vi "GUI_laptop v11g2.vi"() -> ()   [LabVIEW 2019]
uses:
  <vilib>/Math Plots/3D Math Plots/3D Scatter/3D Scatter XCtrl/3D Scatter.xctl
  <vilib>/Platform/TimedLoop/XDataNode/timing_clust.ctl
  <vilib>/Platform/TimedLoop/XDataNode/nitl_modes.ctl
  <vilib>/Platform/TimedLoop/XDataNode/wakeup.ctl
  <vilib>/Analysis/_algsub.llb/Real Vector Norm.vi
  <vilib>/Instr/_visa.llb/VISA Configure Serial Port (Instr).vi
  <vilib>/Utility/file.llb/Write Delimited Spreadsheet (DBL).vi
  <vilib>/addons/System Identification/Data Preprocess.llb/SI Lowpass Filter (MISO Array).vi
  <vilib>/Math Plots/3D Math Plots/3D Scatter/3D Scatter Datatype/Public/Plot Helper (Vector).vi
  <vilib>/platform/TimedLoop/XDataNode/XDataNode.xnode
  <vilib>/Platform/TimedLoop/XDataNode/XDNodeRunTimeDep.lvlib
  <vilib>/Analysis/NI_AALPro.lvlib
  <vilib>/Math Plots/3D Math Plots/3D Scatter/3D Scatter Datatype/3D Scatter Datatype.lvclass
  <vilib>/addons/System Identification/NI_SysID.lvlib
panel:
  in  "l3_init":dbl=2.0
  in  "Motion scale L3 outside rcm":dbl=2.0
  in  "L5 Deadzone":dbl
  in  "Sample rate":u32=500
  in  "Cutoff Frequency":dbl=10.0
  in  "Motion scale L1 L2":dbl=10.0
  in  "Motion scale L3":dbl=2.0
  in  "Save Path 4":path=path "C:/Users/jimmy/Documents/GitHub/Arduino-LabVIEW/zhantao/read_data_abs_filtered.csv"
  in  "Save Path 3":path=path "C:/Users/jimmy/Documents/GitHub/Arduino-LabVIEW/zhantao/read_data_abs_sending.csv"
  out "stimulus signals out":dbl[][](array[numeric]) format="%.2f"
  in  "L5 Offset":dbl
  in  "L5 Scale":dbl=1.0
  in  "Motion Scale L4":dbl=30.0
  out "spreadsheet string":string
  in  "Save Path 2":path=path "C:/Users/jimmy/Documents/GitHub/Arduino-LabVIEW/zhantao/read_data_delt.csv"
  out "send values":dbl[](array[numeric])
  out "Robot Feedback (l1 l2 l3 l4)":dbl[](array[numeric])
  in  "UDP Send":bool
  in  "UDP Recv":bool
  in  "L5 bound":dbl=1000.0
  in  "L4 bound (deg)":dbl=1000.0
  in  "L3 bound (mm)":dbl=1000.0
  in  "L2 bound (deg)":dbl=1000.0
  in  "L1 bound (deg)":dbl=1000.0
  in  "Joystick Type":dbl(ring)=1.0 items=["Rigid Joystick", "Free Joystick"]
  out "Finished Late? [i-1]":bool
  in  "Epsilon":dbl=0.2
  out "3D Scatter":refnum<class "3D Plot Datatype.lvclass">[](xcontrol)
  out "Random Point":dbl[](array[numeric])
  out "Virtual Cursor":dbl[](array[numeric])
  out "Iteration Duration":i64
  in  "Num of Points":i32=10
  in  "z bound":dbl=2.0
  in  "y bound":dbl=5.0
  in  "x bound":dbl=5.0
  in  "Stop":bool
  in  "Round Decimals":dbl=2.0 format="%#_15g"
  in  "Save Data":bool
  in  "Save Path":path=path "C:/Users/jimmy/Documents/GitHub/Arduino-LabVIEW/zhantao/read_data_abs.csv"
  in  "x speed":dbl=0.5
  in  "z speed":dbl=0.5
  in  "y speed":dbl=0.5
  out "error out":errorcluster
  in  "baud rate":u32=250000
  in  "VISA resource name":refnum<visa-resource-name>
  # "Joystick Selection"
  # "Plotting"
  # "Data Saving"
  # "Arduino Communication"
  # "Master Slave Communication"
  # "Parameters"
  # "TODO: add a lowpass filter for l5"
  # "TODO: fix the bounds; currently bounds are arbitrary"
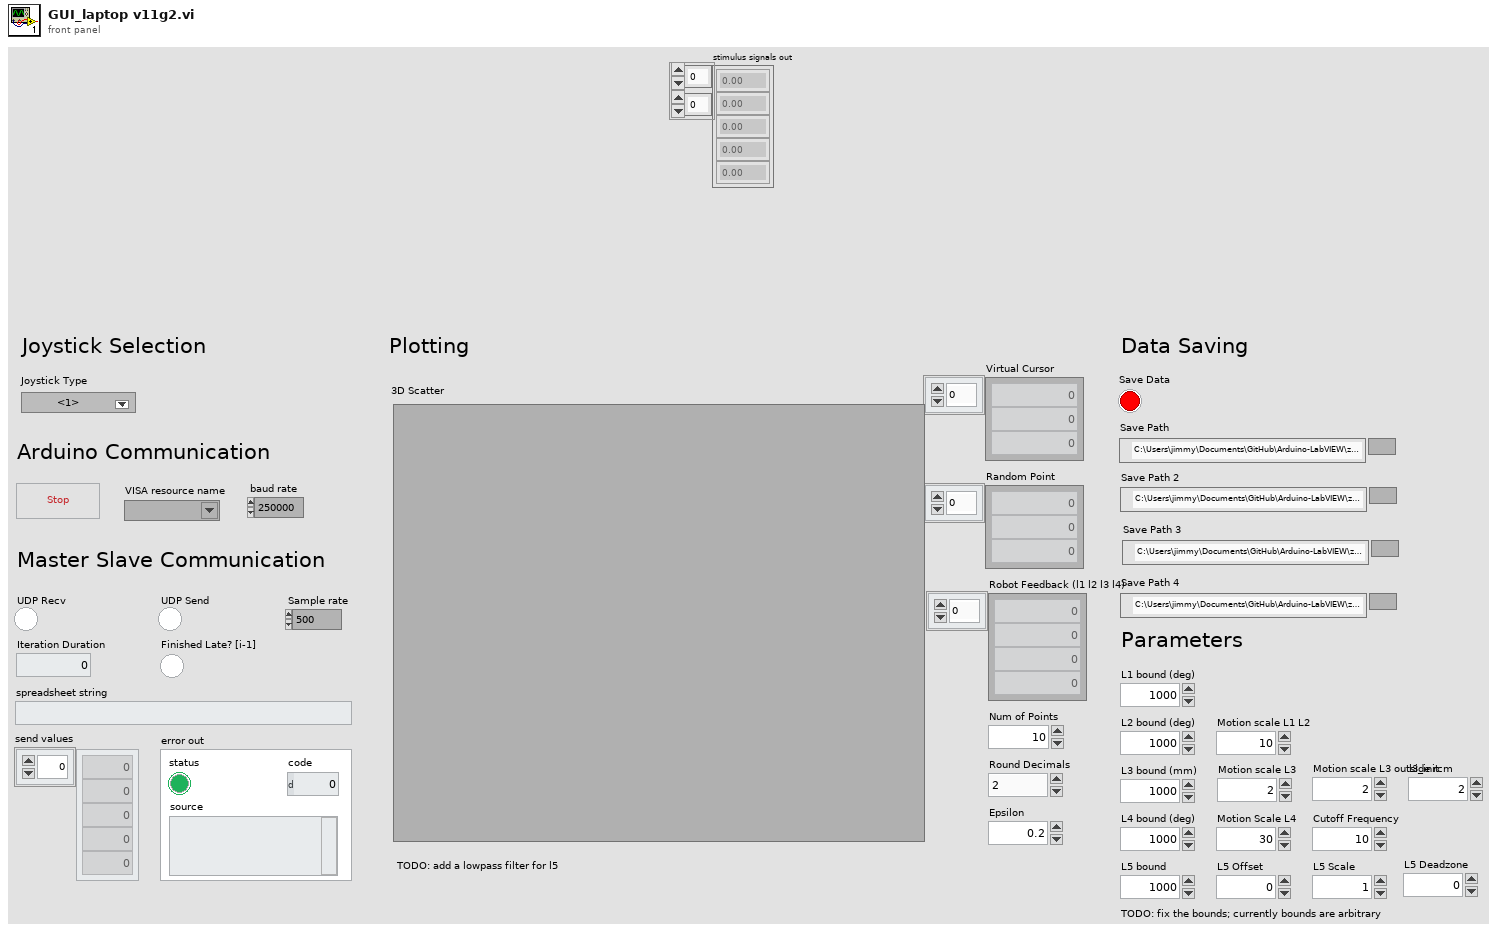
[diagram p1: front panel]
types:
  T1 = typedef "XDNodeRunTimeDep.lvlib/timing_clust.ctl" = cluster{"Expected End [f-1]":u64, "Actual End [f-1]":u64, "Finished Late? [f-1]":bool, "Expected End [i-1]":u64, "Actual End [i-1]":u64, "Finished Late? [i-1]":bool, "Expected Start [i]":u64, "Actual Start [i]":u64, "Expected Start [f]":u64, "Actual Start [f]":u64, "Source Name":string, "Structure Name":string, "Period":i64, "Deadline":i64, "Offset":i64, "Start":i64, "Priority":i32, "Timeout":i32, "Mode":T2, "Wakeup Reason":T3, "Error":errorcluster, "Source Type":string, "Secondary Source Type":string, "Global End Time":u64, "Global Start Time":u64, "Frame Duration":u64, "Iteration Duration":u64, "Assigned CPU":i32, "I/O Scan Engine Mode":u32}
  T2 = typedef "XDNodeRunTimeDep.lvlib/nitl_modes.ctl" = enum32{"No Change", "Process missed periods, maintain original phase", "Discard missed periods, maintain original phase", "Process missed periods, ignore original phase", "Discard missed periods, ignore original phase"}
  T3 = typedef "XDNodeRunTimeDep.lvlib/wakeup.ctl" = enum32{"Normal", "Aborted", "Asynchronous wakeup", "Timing source error", "Timed loop error", "Timeout"}
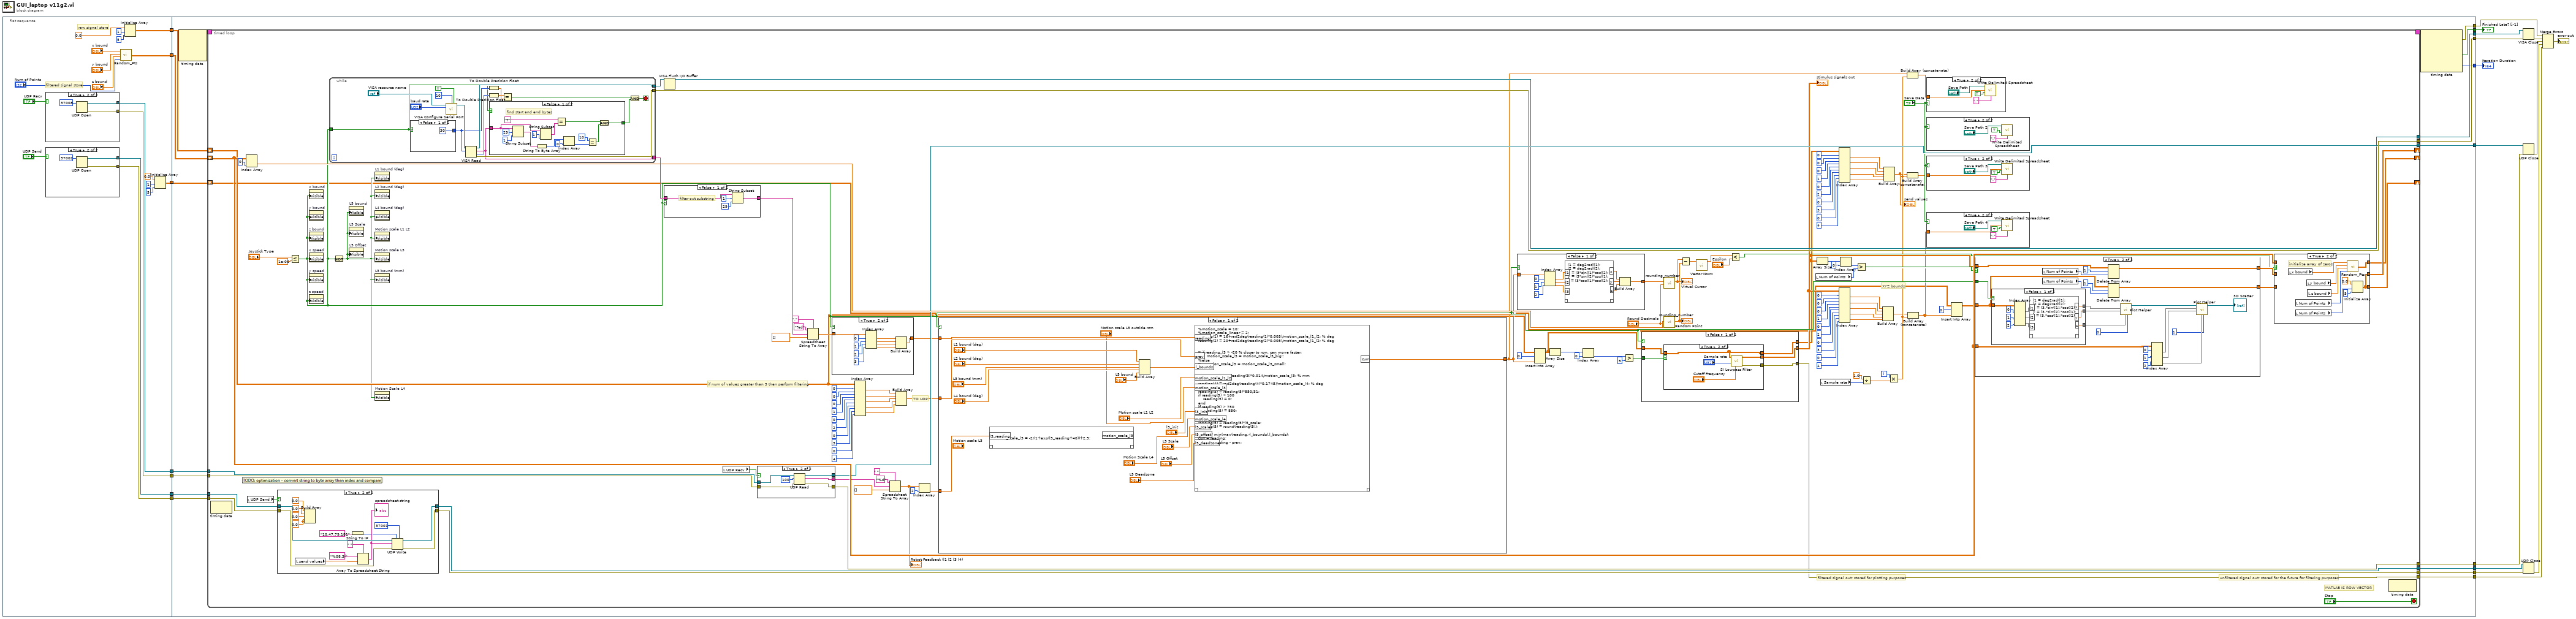
[diagram p0: block diagram]
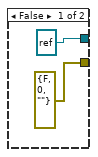
[diagram p2: hidden frame]
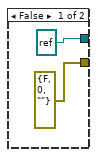
[diagram p3: hidden frame]
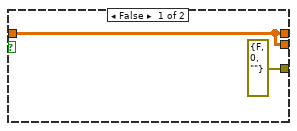
[diagram p6: hidden frame]
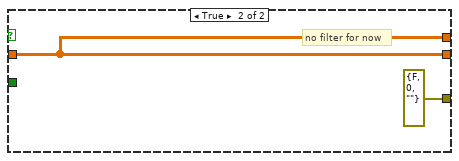
[diagram p7: hidden frame]
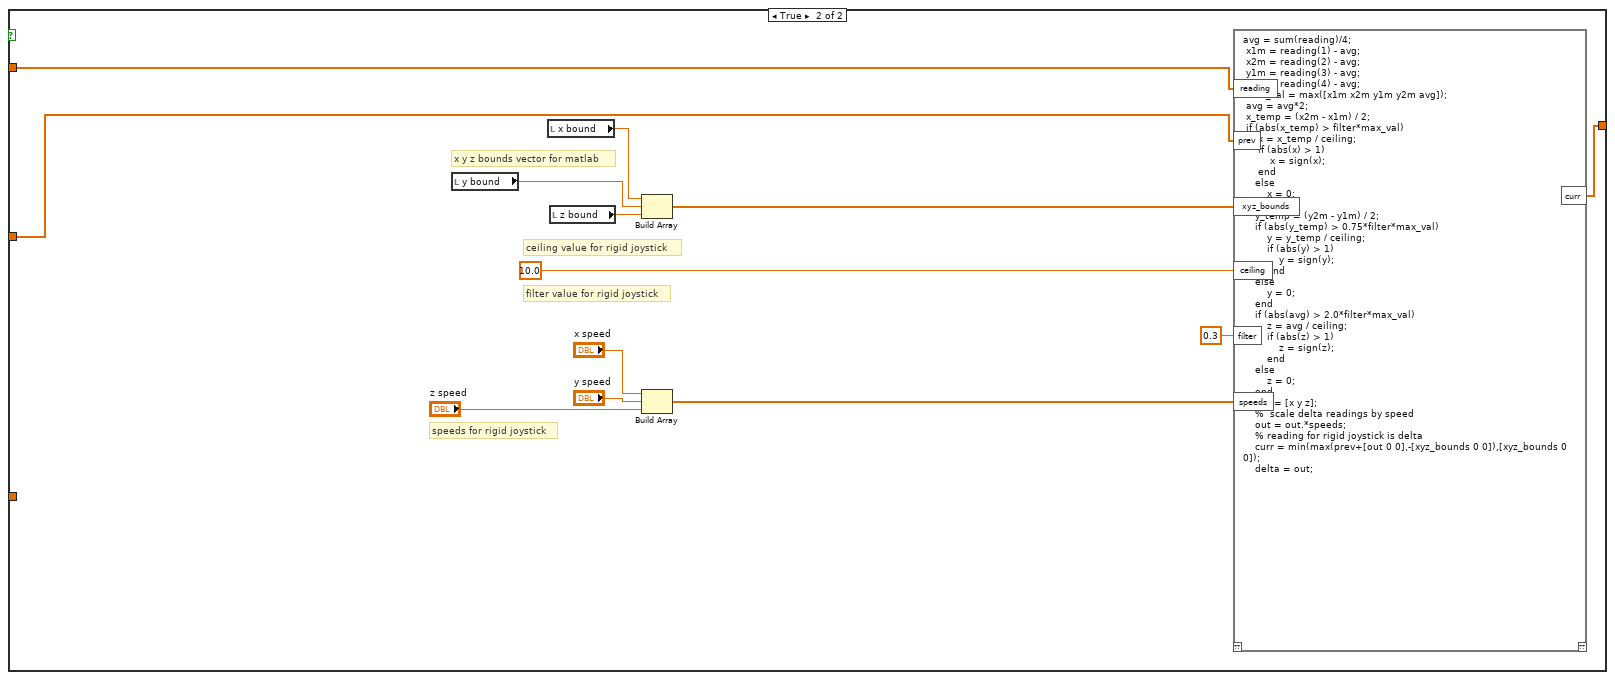
[diagram p8: hidden frame]
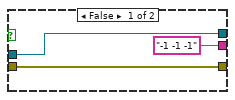
[diagram p11: hidden frame]
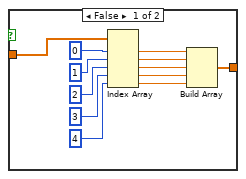
[diagram p15: hidden frame]
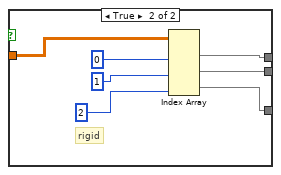
[diagram p18: hidden frame]
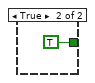
[diagram p19: hidden frame]
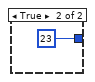
[diagram p20: hidden frame]
diagram:
  n1 = flat-sequence {
    tunnel: [w32] -> w17
    tunnel: [w36] -> w16
    tunnel: [w31] -> w15
    tunnel: [w30] -> w14
    tunnel: [w27] -> w13
    tunnel: [w26] -> w12
    tunnel: [w22] -> w1
    tunnel: [w67] -> w21
    tunnel: [w66] -> w20
    tunnel: [w64] -> w11
    tunnel: [w62] -> w19
    tunnel: [w61] -> w18
    tunnel: w17 -> [w65]
    tunnel: w16 -> [w63]
    tunnel: w15 -> [w60]
    tunnel: w14 -> [w59]
    tunnel: w13 -> [w58]
    tunnel: w12 -> [w57]
    tunnel: [w56] -> w5
    tunnel: [w55] -> w10
    tunnel: [w54] -> w4
    tunnel: [w53] -> w3
    tunnel: [w52] -> w2
    tunnel: w1 -> [w51]
    frame #0 {
      # "filtered signal store"
      # "raw signal store"
      n2 = case shown="True" "UDP Recv" {
        tunnel: [refnum<k16> refnum ("port") w49] -> w30
        tunnel: [errorcluster {"status"=FALSE, "code"=0, "source"=""} ("error out") w48] -> w27
        frame False {
        }
        frame True {
          n3 = UDP Open(11:u16 37008 ("port")) -> (port=w49:refnum<k16>, 0:w48:errorcluster)  [unwired: 4 in, 1 out]
        }
      }
      n4 = case shown="True" "UDP Send" {
        tunnel: [refnum<k16> refnum ("port") w44] -> w31
        tunnel: [errorcluster {"status"=FALSE, "code"=0, "source"=""} ("error out") w43] -> w26
        frame False {
        }
        frame True {
          n5 = UDP Open(11:u16 37002 ("port")) -> (port=w44:refnum<k16>, 0:w43:errorcluster)  [unwired: 4 in, 1 out]
        }
      }
      n6 = call "Random_Pts.vi"("Num of Points"="Num of Points", "z bound"="z bound", "y bound"="y bound", "x bound"="x bound") -> ("appended array"=w36:dbl[][])
      n7 = Initialize Array(0.0 ("element"), 1 ("dimension size"), 5 ("dimension size")) -> (w32:dbl[][])
      n8 = Initialize Array(0.0 ("element"), 1 ("dimension size"), 5 ("dimension size")) -> (w22:dbl[][])
    }
    frame #1 {
      n9 = node-c288() -> (w69:T1)  [unwired: 4 in]
      n10 = timed-loop {
        tunnel: [w137] -> w67
        tunnel: [w193] -> w66
        shift-right: [w192] -> _
        shift-left: w65 -> [w91]
        timing: w69 -> [_]
        timing-out: [_] -> w68
        shift-right: [w188] -> _
        shift-left: w63 -> [w189]
        tunnel: w60 -> [w151]
        tunnel: w59 -> [w150]
        tunnel: w58 -> [w148]
        tunnel: w57 -> [w147]
        tunnel: [w146] -> w56
        tunnel: [w145] -> w55
        tunnel: [w144] -> w54
        tunnel: [w143] -> w53
        tunnel: [w126] -> w52
        shift-right: [w82] -> _
        shift-left: w51 -> [w85]
        i -> [w80]
        stop <- "Stop" stop-if-true
        # "unfiltered signal out; stored for the future for filtering purposes"
        # "filtered signal out; stored for plotting purposes"
        # "XYZ bounds"
        # "if num of values greater than 5 then perform filtering"
        # "TO UDP"
        # "MATLAB IS ROW VECTOR"
        n11 = node-c288() -> ()  [unwired: 1 in, 1 out]
        n12 = Index Array(array=w189, index (col)=0 ("index (row)")) -> (element=w160:dbl[])  [unwired: 1 in]
        n13 = local read "UDP Send"() -> (w75:bool)
        n14 = case shown="True" w75 {
          tunnel: w151 -> [w250 w266]
          tunnel: w147 -> [w251 w262]
          tunnel: [w251 w258] -> w145
          tunnel: [w250 w257] -> w143
          frame False {
          }
          frame True {
            w256 = 0.0 ("element")
            n15 = local read "send values"() -> (w252:dbl[])
            n16 = Build Array(0.0 ("element"), 0.0 ("element"), 0.0 ("element"), w256, w256) -> ()  [unwired: 1 out]
            n17 = String To IP(1:"10.47.79.181" ("name")) -> (0:w260:u32)
            n18 = Array To Spreadsheet String(delimiter (Tab)=" ", array=w252, 3:"%08.3f" ("format string")) -> (spreadsheet string=w263:string)
            "spreadsheet string" <- w263
            n19 = UDP Write(address=w260, port or service name=u16 37001, connection ID=w266, data in=w263, 8:w262) -> (error out=w258:errorcluster, 3:w257:refnum<k16>)  [unwired: 1 in]
          }
        }
        n20 = Less Or Equal?(x="Joystick Type", y=1e-06) -> (x <= y?=w127:bool)
        n21 = property on="x bound" class="DigNum (strict)"("Visible"=w127) -> ()  [unwired: 2 in, 2 out]
        n22 = property on="y bound" class="DigNum (strict)"("Visible"=w127) -> ()  [unwired: 2 in, 2 out]
        n23 = property on="z bound" class="DigNum (strict)"("Visible"=w127) -> ()  [unwired: 2 in, 2 out]
        n24 = property on="x speed" class="DigNum (strict)"("Visible"=w127) -> ()  [unwired: 2 in, 2 out]
        n25 = property on="y speed" class="DigNum (strict)"("Visible"=w127) -> ()  [unwired: 2 in, 2 out]
        n26 = property on="z speed" class="DigNum (strict)"("Visible"=w127) -> ()  [unwired: 2 in, 2 out]
        n27 = while {
          tunnel: [w373] -> w162
          tunnel: [w386] -> w193
          tunnel: [w380] -> w138
          tunnel: w127 -> [w374]
          stop <- w376 stop-if-true
          n28 = case shown="False" w374 {
            tunnel: [30 u32 23 ("byte count")] -> w379
            frame False {
            }
            frame True {
            }
          }
          n29 = call-poly "VISA Configure Serial Port"("VISA resource name"="VISA resource name", "termination char\n(0xA = '\\n' = LF)"=u8 10 ("termination char\n(0xA = '\\n' = LF)"), "Enable Termination\nChar (T)"=TRUE ("Enable Termination\nChar (T)"), "baud rate (9600)"="baud rate") -> ("VISA resource name out"=w381:refnum<visa-resource-name>)  [unwired: 10 in, 1 out]
          n30 = VISA Read(VISA resource name=w381, byte count=w379) -> (VISA resource name out=w380:refnum<visa-resource-name>, read buffer=w373:string, return count=w388:u32, error out=w386:errorcluster)  [unwired: 1 in]
          n31 = To Double Precision Float(number=w379) -> (double precision float=w378:dbl)
          n32 = To Double Precision Float(number=w388) -> (double precision float=w387:dbl)
          n33 = case shown="False" w374 {
            tunnel: [w395 TRUE] -> w375
            tunnel: w373 -> [w398 _]
            frame False {
              # "find start and end bytes"
              n34 = String Subset(string=w398, offset (0)=29, length (rest)=1) -> (substring=w393:string)
              n35 = String To Byte Array(string=w393) -> (unsigned byte array=w392:u8[])
              n36 = String Subset(string=w398, length (rest)=1) -> (substring=w401:string)  [unwired: 1 in]
              n37 = Equal?(x="T", y=w401) -> (x = y?=w397:bool)
              n38 = Index Array(array=w392, index=0) -> (element=w390:u8)
              n39 = Equal?(x=10, y=w390) -> (x = y?=w396:bool)
              n40 = And(x=w397, y=w396) -> (x .and. y?=w395:bool)
            }
            frame True {
            }
          }
          n41 = Equal?(x=w387, y=w378) -> (x = y?=w377:bool)
          n42 = And(x=w377, y=w375) -> (x .and. y?=w376:bool)
        }
        n43 = Not(x=w127) -> (.not. x?=w89:bool)
        n44 = property on="L5 bound" class="DigNum (strict)"("Visible"=w89) -> ()  [unwired: 2 in, 2 out]
        n45 = property on="L5 Scale" class="DigNum (strict)"("Visible"=w89) -> ()  [unwired: 2 in, 2 out]
        n46 = property on="L5 Offset" class="DigNum (strict)"("Visible"=w89) -> ()  [unwired: 2 in, 2 out]
        n47 = property on="L1 bound (deg)" class="DigNum (strict)"("Visible"=w89) -> ()  [unwired: 2 in, 2 out]
        n48 = property on="L2 bound (deg)" class="DigNum (strict)"("Visible"=w89) -> ()  [unwired: 2 in, 2 out]
        n49 = property on="L4 bound (deg)" class="DigNum (strict)"("Visible"=w89) -> ()  [unwired: 2 in, 2 out]
        n50 = property on="Motion scale L1 L2" class="DigNum (strict)"("Visible"=w89) -> ()  [unwired: 2 in, 2 out]
        n51 = property on="Motion scale L3" class="DigNum (strict)"("Visible"=w89) -> ()  [unwired: 2 in, 2 out]
        n52 = property on="L3 bound (mm)" class="DigNum (strict)"("Visible"=w89) -> ()  [unwired: 2 in, 2 out]
        n53 = property on="Motion Scale L4" class="DigNum (strict)"("Visible"=w89) -> ()  [unwired: 2 in, 2 out]
        n54 = VISA Flush I/O Buffer(VISA resource name=w138) -> (VISA resource name out=w137:refnum<visa-resource-name>)  [unwired: 2 in, 1 out]
        n55 = case shown="False" w127 {
          tunnel: w162 -> [w295 w296]
          tunnel: [w292 w296] -> w161
          frame False {
            # "filter out substring"
            n56 = String Subset(string=w295, offset (0)=1, length (rest)=29) -> (substring=w292:string)
          }
          frame True {
          }
        }
        n57 = local read "UDP Recv"() -> (w149:bool)
        n58 = case shown="True" w149 {
          tunnel: w150 -> [w268 w275]
          tunnel: w148 -> [w269 w274]
          tunnel: [w269 w273] -> w146
          tunnel: [w268 w272] -> w144
          tunnel: ["-1 -1 -1" w270] -> w139
          frame False {
          }
          frame True {
            n59 = UDP Read(connection ID=w275, max size (548)=100, 8:w274) -> (data out=w270:string, error out=w273:errorcluster, 3:w272:refnum<k16>)  [unwired: 1 in, 2 out]
          }
        }
        n60 = Spreadsheet String To Array(delimiter (Tab)=",", format string="%d", spreadsheet string=w161, array type (2D Dbl)=dbl[] []) -> (array=w163:dbl[])
        n61 = case shown="True" w127 {
          tunnel: w163 -> [w297 w312]
          tunnel: [w302 w311] -> w135
          frame False {
            n62 = Index Array(array=w297, index #1=0 ("Plot ID"), index #2=1 ("Plot ID"), index #3=2 ("Plot ID"), index #4=3 ("Plot ID"), index #5=4 ("Plot ID")) -> (element #1=w305:dbl, element #2=w304:dbl, element #3=w303:dbl, element #4=w299:dbl, element #5=w298:dbl)
            n63 = Build Array(w305, w304, w303, w299, w298) -> (w302:dbl[])
          }
          frame True {
            n64 = Index Array(array=w312, index #1=0 ("Plot ID"), index #2=1 ("Plot ID"), index #3=2 ("Plot ID"), index #4=3 ("index")) -> (element #1=w315:dbl, element #2=w314:dbl, element #3=w313:dbl, element #4=w309:dbl)
            n65 = Build Array(w315, w314, w313, w309) -> (w311:dbl[])
          }
        }
        n66 = Index Array(array=w91, index (row) #1=0 ("disabled index (row)"), index (col) #1=0 ("disabled index (col)"), index (row) #2=0 ("disabled index (row)"), index (col) #2=1 ("disabled index (col)"), index (row) #3=0 ("disabled index (row)"), index (col) #3=2 ("disabled index (col)"), index (row) #4=0 ("disabled index (row)"), index (col) #4=3 ("disabled index (col)"), index (row) #5=0 ("disabled index (row)"), index (col) #5=4 ("disabled index (col)")) -> (element #1=w174:dbl, element #2=w173:dbl, element #3=w172:dbl, element #4=w165:dbl, element #5=w164:dbl)
        n67 = Spreadsheet String To Array(delimiter (Tab)=" ", format string="%d", spreadsheet string=w139, array type (2D Dbl)=dbl[] []) -> (array=w72:dbl[])
        "Robot Feedback (l1 l2 l3 l4)" <- w72
        n68 = Build Array(w174, w173, w172, w165, w164) -> (w136:dbl[])
        n69 = Index Array(array=w72, index=2) -> (element=w70:dbl)
        n70 = case shown="False" w127 {
          tunnel: w136 -> [w225 w236]
          tunnel: w135 -> [w226 w235]
          tunnel: [w224 w234] -> w110
          tunnel: w70 -> [w218 _]
          frame False {
            n71 = script code="motion_scale_l3 = -2/(1+exp(l3_reading+40))+2.5;"("l3_reading"=w218) -> ()  [unwired: 1 in, 2 out]
            n72 = Build Array("L1 bound (deg)", "L2 bound (deg)", "L3 bound (mm)", "L4 bound (deg)", "L5 bound") -> (w227:dbl[])
            n73 = script code="%motion_scale = 10;\n%motion_scale_linear = 2;\nreading(1) = 16+rad2deg(reading(1)*0.005)/motion_scale_l1_l2; % deg\nreading(2) = 20+rad2deg(reading(2)*0.005)/motion_scale_l1_l2; % deg\n\n\n%if reading_l3 > -20 % closer to rcm, can move faster;\n%    motion_scale_l3 = motion_scale_l3_big;;\n%else\n%   motion_scale_l3 = motion_scale_l3_small;\n%end\n\nreading(3) = -40-reading(3)*0.014/motion_scale_l3; % mm\n\nreading(4) = rad2deg(reading(4)*0.1745)/motion_scale_l4; % deg\n\nreading(5) = reading(5)*850/31;\nif reading(5) < 100\n    reading(5) = 0;\nend\nif reading(5) > 750\n    reading(5) = 850;\nend\n\nreading(5) = reading(5)*l5_scale;\nreading(5) = round(reading(5));\n\n%curr = min(max(reading,-l_bounds),l_bounds);\ncurr = reading;\ndelta = reading - prev;"("l_bounds"=w227, "motion_scale_l4"="Motion Scale L4", "reading"=w226, "prev"=w225, "l5_scale"="L5 Scale", "l5_offset"="L5 Offset", "motion_scale_l3"="Motion scale L3 outside rcm", "motion_scale_l1_l2"="Motion scale L1 L2", "l5_deadzone"="L5 Deadzone", "l3_init"="l3_init") -> ("curr"=w224:dbl[])  [unwired: 1 in, 1 out]
          }
          frame True {
            # "ceiling value for rigid joystick"
            # "filter value for rigid joystick"
            # "speeds for rigid joystick"
            # "x y z bounds vector for matlab"
            n74 = local read "y bound"() -> (w245:dbl)
            n75 = local read "x bound"() -> (w244:dbl)
            n76 = local read "z bound"() -> (w246:dbl)
            n77 = Build Array(w244, w245, w246) -> (w237:dbl[])
            n78 = Build Array("x speed", "y speed", "z speed") -> (w240:dbl[])
            n79 = script code="avg = sum(reading)/4;\n x1m = reading(1) - avg;\n x2m = reading(2) - avg;\n y1m = reading(3) - avg;\n y2m = reading(4) - avg;\n max_val = max([x1m x2m y1m y2m avg]);\n avg = avg*2;\n x_temp = (x2m - x1m) / 2;\n if (abs(x_temp) > filter*max_val)\n     x = x_temp / ceiling;\n     if (abs(x) > 1)\n         x = sign(x);\n     end\n    else\n        x = 0;\n    end\n    y_temp = (y2m - y1m) / 2;\n    if (abs(y_temp) > 0.75*filter*max_val)\n        y = y_temp / ceiling;\n        if (abs(y) > 1)\n            y = sign(y);\n        end\n    else\n        y = 0;\n    end\n    if (abs(avg) > 2.0*filter*max_val)\n        z = avg / ceiling;\n        if (abs(z) > 1)\n            z = sign(z);\n        end\n    else\n        z = 0;\n    end\n    out = [x y z];\n    %  scale delta readings by speed\n    out = out.*speeds;\n    % reading for rigid joystick is delta\n    curr = min(max(prev+[out 0 0],-[xyz_bounds 0 0]),[xyz_bounds 0 0]);\n    delta = out;"("xyz_bounds"=w237, "ceiling"=10.0 ("Real"), "filter"=0.3 ("Real"), "speeds"=w240, "reading"=w235, "prev"=w236) -> ("curr"=w234:dbl[])  [unwired: 1 in, 1 out]
          }
        }
        n80 = case shown="False" w127 {
          tunnel: [w323 w330] -> w190
          tunnel: w110 -> [w322 w330]
          frame False {
            n81 = Index Array(array=w322, index #1=0 ("Plot ID"), index #2=1 ("Plot ID"), index #3=2 ("Plot ID")) -> (element #1=w321:dbl, element #2=w320:dbl, element #3=w319:dbl)
            n82 = script code="l1 = deg2rad(l1);\nl2 = deg2rad(l2);\nx = l3*sin(l1)*cos(l2);\ny = l3*sin(l2)*cos(l1);\nz = l3*cos(l1)*cos(l2);"("l1"=w321, "l2"=w320, "l3"=w319) -> ("x"=w326:dbl, "y"=w325:dbl, "z"=w324:dbl)  [unwired: 1 in, 1 out]
            n83 = Build Array(w326, w325, w324) -> (w323:dbl[])
          }
          frame True {
          }
        }
        n84 = Insert Into Array(array=w91, index (row)=0, new element=w110) -> (w128:dbl[][])  [unwired: 1 in]
        n85 = Array Size(array=w128) -> (size(s)=w131:i32[])
        n86 = Index Array(array=w131, index=0) -> (element=w130:i32)
        n87 = Greater?(x=w130, y=5) -> (0:w76:bool)
        n88 = case shown="False" w127 {
          tunnel: w76 -> [w205 _]
          tunnel: w128 -> [w207 w215]
          tunnel: [w206 w215] -> w88
          tunnel: [w204 errorcluster {"status"=FALSE, "code"=0, "source"=""} ("error out")] -> w126
          tunnel: [w203 w215] -> w92
          frame False {
            n89 = case shown="True" w205 {
              tunnel: w207 -> [w208 w213]
              tunnel: [w208 w213] -> w206
              tunnel: [errorcluster {"status"=FALSE, "code"=0, "source"=""} ("error out") w214] -> w204
              tunnel: [w208 w212] -> w203
              frame False {
              }
              frame True {
                n90 = call-poly <vilib>:"SI Lowpass Filter.vi"("cutoff frequency"="Cutoff Frequency", "sampling rate (Hz)"="Sample rate", "stimulus signals in"=w213) -> ("error out"=w214:errorcluster, "stimulus signals out"=w212:dbl[][])  [unwired: 6 in, 1 out]
              }
            }
          }
          frame True {
            # "no filter for now"
          }
        }
        "stimulus signals out" <- w92
        n91 = call "rounding_number.vi"("power of ten"="Round Decimals", "Array"=w190) -> ("rounded"=w158:dbl[])  [unwired: 9 in]
        "Virtual Cursor" <- w158
        n92 = call "rounding_number.vi"("power of ten"="Round Decimals", "Array"=w160) -> ("rounded"=w157:dbl[])  [unwired: 9 in]
        "Random Point" <- w157
        n93 = Subtract(x=w158, y=w157) -> (x-y=w156:dbl[])
        n94 = call-poly <vilib>:"Vector Norm.vi"("Input Vector"=w156) -> ("norm"=w155:dbl)  [unwired: 9 in, 1 out]
        n95 = Less?(x=w155, y="Epsilon") -> (x < y?=w153:bool)
        n96 = local read "Num of Points"() -> (w176:i32)
        n97 = Array Size(array=w88) -> (size(s)=w134:i32[])
        n98 = local read "Sample rate"() -> (w77:u32)
        n99 = Index Array(array=w88, index (row) #1=0 ("disabled index (col)"), index (col) #1=0 ("disabled index (row)"), index (row) #2=0 ("disabled index (col)"), index (col) #2=1 ("disabled index (row)"), index (row) #3=0 ("disabled index (col)"), index (col) #3=2 ("disabled index (row)"), index (row) #4=0 ("disabled index (col)"), index (col) #4=3 ("disabled index (row)"), index (row) #5=0 ("disabled index (col)"), index (col) #5=4 ("disabled index (col)")) -> (element #1=w115:dbl, element #2=w114:dbl, element #3=w113:dbl, element #4=w112:dbl, element #5=w111:dbl)
        n100 = Index Array(array=w92, index (row) #1=0 ("disabled index (col)"), index (col) #1=0 ("disabled index (row)"), index (row) #2=0 ("disabled index (col)"), index (col) #2=1 ("disabled index (row)"), index (row) #3=0 ("disabled index (col)"), index (col) #3=2 ("disabled index (row)"), index (row) #4=0 ("disabled index (col)"), index (col) #4=3 ("disabled index (row)"), index (row) #5=0 ("disabled index (col)"), index (col) #5=4 ("disabled index (col)")) -> (element #1=w98:dbl, element #2=w97:dbl, element #3=w96:dbl, element #4=w95:dbl, element #5=w94:dbl)
        n101 = Index Array(array=w134, index=0) -> (element=w177:i32)
        n102 = Greater?(x=w177, y=w176) -> (0:w175:bool)
        n103 = Divide(x=1.0, y=w77) -> (x/y=w78:dbl)
        n104 = Build Array(w98, w97, w96, w95, w94) -> (w74:dbl[])
        n105 = Build Array(w115, w114, w113, w112, w111) -> (w73:dbl[])
        "send values" <- w73
        n106 = Multiply(x=w80, y=w78) -> (x*y=w81:dbl)
        n107 = Build Array (concatenate)(w110, w81) -> (w109:dbl[])
        n108 = Build Array (concatenate)(w73, w81) -> (w90:dbl[])
        n109 = Build Array (concatenate)(w74, w81) -> (w86:dbl[])
        n110 = case shown="True" "Save Data" {
          tunnel: w109 -> [_ w276]
          frame False {
          }
          frame True {
            n111 = call-poly <vilib>:"Write Delimited Spreadsheet.vi"("file path (dialog if empty)"="Save Path", "1D data"=w276, "append to file? (new file:F)"=TRUE, "delimiter (\\t)"="," ("delimiter (\\t)")) -> ()  [unwired: 10 in, 2 out]
          }
        }
        n112 = case shown="True" "Save Data" {
          frame False {
          }
          frame True {
            n113 = call-poly <vilib>:"Write Delimited Spreadsheet.vi"("file path (dialog if empty)"="Save Path 2", "append to file? (new file:F)"=TRUE, "delimiter (\\t)"="," ("delimiter (\\t)")) -> ()  [unwired: 11 in, 2 out]
          }
        }
        n114 = case shown="True" "Save Data" {
          tunnel: w90 -> [_ w199]
          frame False {
          }
          frame True {
            n115 = call-poly <vilib>:"Write Delimited Spreadsheet.vi"("file path (dialog if empty)"="Save Path 3", "1D data"=w199, "append to file? (new file:F)"=TRUE, "delimiter (\\t)"="," ("delimiter (\\t)")) -> ()  [unwired: 10 in, 2 out]
          }
        }
        n116 = case shown="True" "Save Data" {
          tunnel: w86 -> [_ w195]
          frame False {
          }
          frame True {
            n117 = call-poly <vilib>:"Write Delimited Spreadsheet.vi"("file path (dialog if empty)"="Save Path 4", "1D data"=w195, "append to file? (new file:F)"=TRUE, "delimiter (\\t)"="," ("delimiter (\\t)")) -> ()  [unwired: 10 in, 2 out]
          }
        }
        n118 = Insert Into Array(array=w85, index (row)=0, new element=w86) -> (w84:dbl[][])  [unwired: 1 in]
        n119 = case shown="True" w175 {
          tunnel: w88 -> [w332 w354]
          tunnel: [w332 w353] -> w191
          tunnel: w189 -> [w331 w352]
          tunnel: w127 -> [_ w337]
          tunnel: w84 -> [_ w334]
          tunnel: [w331 w333] -> w83
          frame False {
          }
          frame True {
            n120 = case shown="False" w337 {
              tunnel: w334 -> [w365 w369]
              tunnel: [w356 w368] -> w343
              tunnel: [w357 w367] -> w342
              tunnel: [w358 w366] -> w341
              frame False {
                n121 = Index Array(array=w365, index (col) #1=0 ("Plot ID"), index (col) #2=1 ("Plot ID"), index (col) #3=2 ("Plot ID")) -> (element #1=w361:dbl[], element #2=w360:dbl[], element #3=w359:dbl[])  [unwired: 3 in]
                n122 = script code="l1 = deg2rad(l1);\nl2 = deg2rad(l2);\nx = l3.*sin(l1).*cos(l2);\ny = l3.*sin(l2).*cos(l1);\nz = l3.*cos(l1).*cos(l2);"("l1"=w361, "l2"=w360, "l3"=w359) -> ("x"=w356:dbl[], "y"=w357:dbl[], "z"=w358:dbl[])  [unwired: 1 in, 1 out]
              }
              frame True {
                # "rigid"
                n123 = Index Array(array=w369, index (col) #1=0 ("disabled index (col)"), index (col) #2=1 ("index (col)"), index (col) #3=2 ("index (col)")) -> (element #1=w368:dbl[], element #2=w367:dbl[], element #3=w366:dbl[])  [unwired: 3 in]
              }
            }
            n124 = local read "Num of Points"() -> (w351:i32)
            n125 = local read "Num of Points"() -> (w336:i32)
            n126 = Delete From Array(array=w354, length=1, index (row)=w351) -> (array with subset deleted=w353:dbl[][])  [unwired: 1 in, 1 out]
            n127 = Delete From Array(array=w334, length=1, index (row)=w336) -> (array with subset deleted=w333:dbl[][])  [unwired: 1 in, 1 out]
            n128 = call-poly <vilib>:"Plot Helper.vi"("Plot ID"=0, "z vector"=w341, "y vector"=w342, "x vector"=w343) -> ("3D Plot lvclass Array out"=w345:refnum<class "3D Plot Datatype.lvclass">[])  [unwired: 2 in, 5 out]
            n129 = Index Array(array=w352, index (row) #1=0 ("index (row)"), index (row) #2=1 ("index (row)"), index (row) #3=2 ("index (row)")) -> (element #1=w349:dbl[], element #2=w348:dbl[], element #3=w347:dbl[])  [unwired: 3 in]
            n130 = call-poly <vilib>:"Plot Helper.vi"("Plot ID"=1, "z vector"=w347, "y vector"=w348, "x vector"=w349, "3D Plot lvclass Array in"=w345) -> ("3D Plot lvclass Array out"=→"3D Scatter":refnum<class "3D Plot Datatype.lvclass">[])  [unwired: 1 in, 5 out]
          }
        }
        n131 = case shown="True" w153 {
          tunnel: w189 -> [w282 _]
          tunnel: [w282 w287] -> w188
          tunnel: w191 -> [w281 _]
          tunnel: [w281 w283] -> w192
          tunnel: w83 -> [w280 _]
          tunnel: [w280 w283] -> w82
          frame False {
          }
          frame True {
            # "initialize array of zeros"
            n132 = local read "x bound"() -> (w291:dbl)
            n133 = local read "Num of Points"() -> (w288:i32)
            n134 = local read "Num of Points"() -> (w285:i32)
            n135 = local read "y bound"() -> (w290:dbl)
            n136 = local read "z bound"() -> (w289:dbl)
            n137 = call "Random_Pts.vi"("Num of Points"=w288, "z bound"=w289, "y bound"=w290, "x bound"=w291) -> ("appended array"=w287:dbl[][])
            n138 = Initialize Array(0.0 ("element"), w285, 5 ("dimension size")) -> (w283:dbl[][])
          }
        }
        n139 = node-c288() -> ()  [unwired: 1 in, 1 out]
      }
      n140 = node-c288(w68) -> (w64:errorcluster, w61:bool, w62:i64)  [unwired: 3 out]
    }
  }
  n141 = VISA Close(VISA resource name=w21, error in (no error)=w20) -> (error out=w9:errorcluster)
  n142 = UDP Close(connection ID=w4, 8:w5) -> (error out=w8:errorcluster)  [unwired: 1 out]
  n143 = UDP Close(connection ID=w3, 8:w10) -> (error out=w7:errorcluster)  [unwired: 1 out]
  n144 = Merge Errors(w11, w9, w8, w7, w2) -> (→"error out":errorcluster)
  "Iteration Duration" <- w19
  "Finished Late? [i-1]" <- w18
